vi "Stop Total Turnos.vi"(8 "error in (no error)":errorcluster, 11 "Manejo Turnos in":refnum<class "Manejo Turnos.lvclass">) -> (0 "error out":errorcluster, 3 "Manejo Turnos out":refnum<class "Manejo Turnos.lvclass">)   [LabVIEW 2020, in "Manejo Turnos.lvlib" / "Manejo Turnos.lvclass"]
uses:
  Manejo Turnos.lvclass
  Manejo Turnos.lvclass/Manejo Turnos.ctl
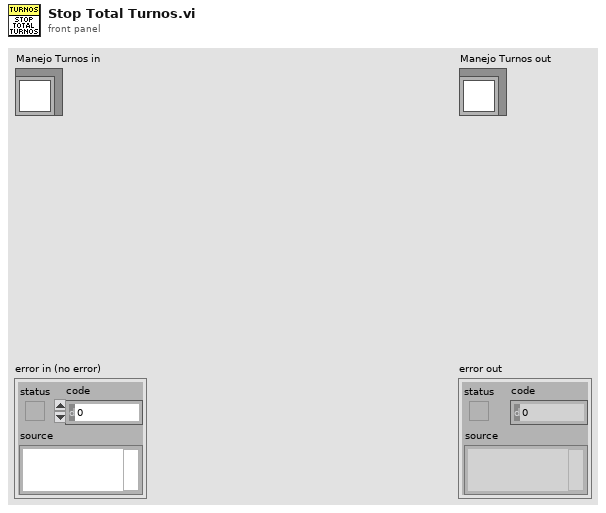
[diagram p1: front panel]
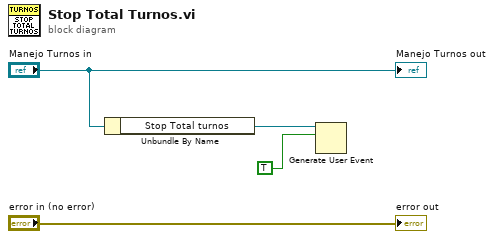
[diagram p0: block diagram]
diagram:
  n1 = Unbundle By Name("Manejo Turnos in") -> ("Stop Total turnos"=w1:refnum<user-event>)
  n2 = Generate User Event(user event=w1, event data cluster=TRUE) -> ()  [unwired: 2 in, 2 out]
  "error out" <- "error in (no error)"
  "Manejo Turnos out" <- "Manejo Turnos in"
